vi "Read_Full.vi"(8 "error in (no error)":errorcluster, 10 "Results Array In":dbl[](array[numeric]), 11 "SoftmotionAxis in":refnum<class "SoftmotionAxis.lvclass">) -> (0 "error out":errorcluster, 2 "appended array":dbl[](array[numeric]), 3 "SoftmotionAxis out":refnum<class "SoftmotionAxis.lvclass">)   [LabVIEW 2017, in "SoftmotionAxis.lvclass"]
uses:
  SoftmotionAxis.lvclass
  <resource>/objmgr/nimcai.rc
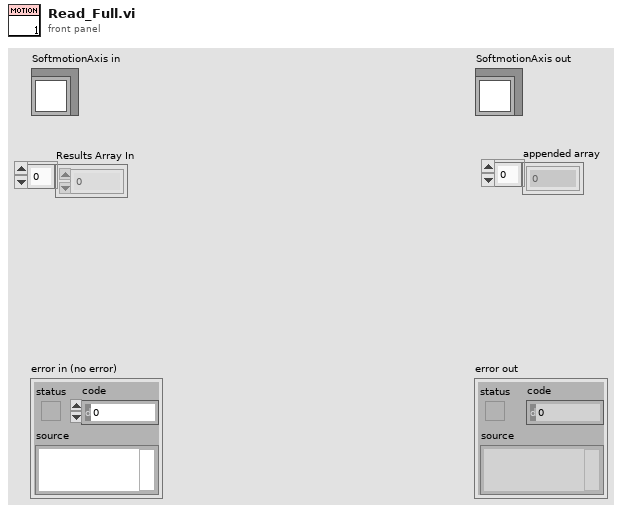
[diagram p1: front panel]
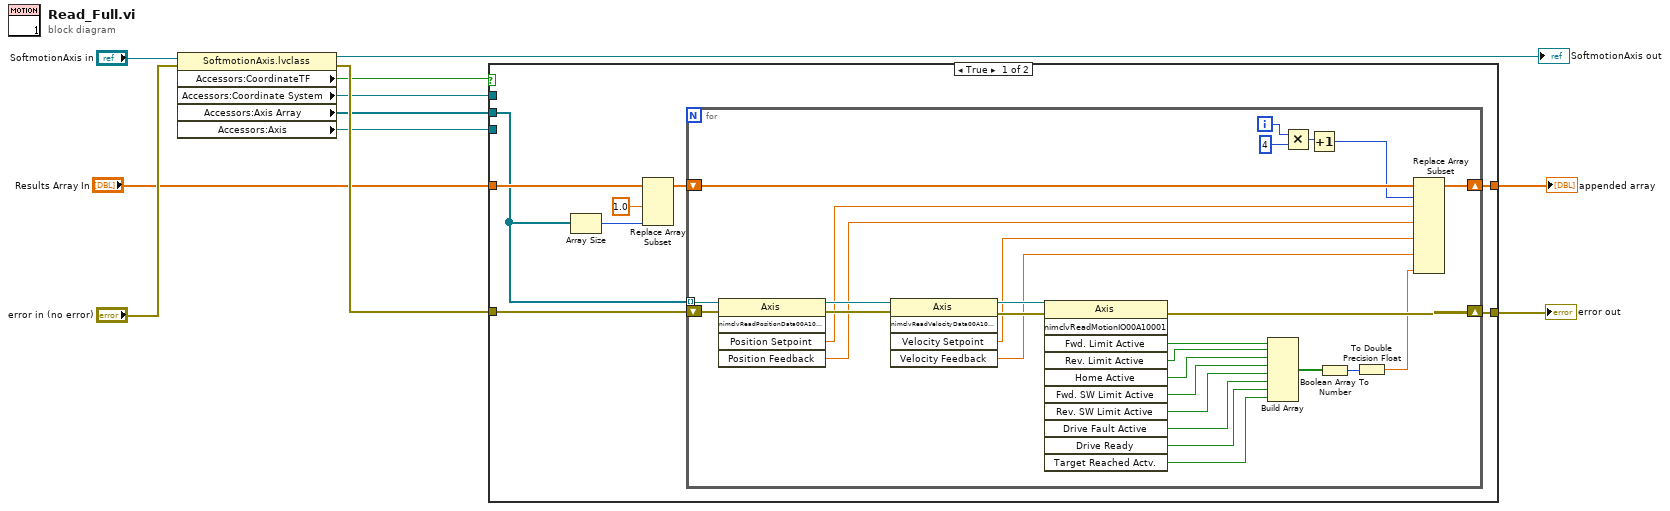
[diagram p0: block diagram]
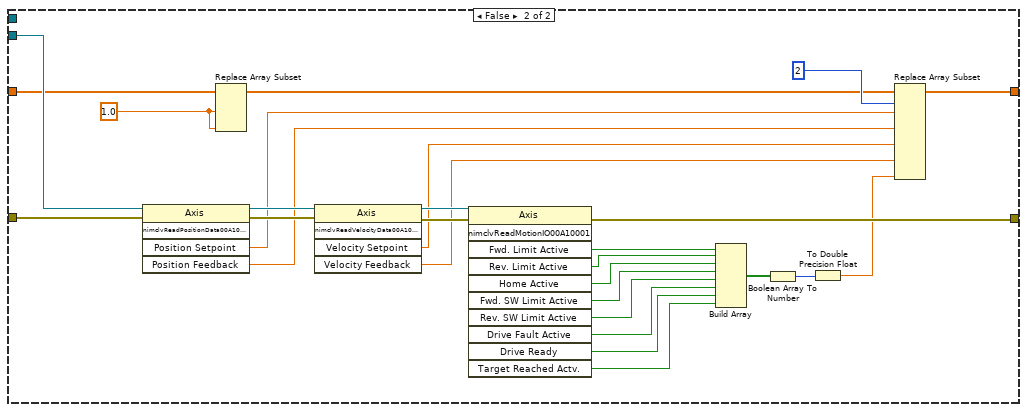
[diagram p2: hidden frame]
diagram:
  n1 = property class="SoftmotionAxis.lvclass"(reference="SoftmotionAxis in", error in="error in (no error)") -> (reference out=→"SoftmotionAxis out":refnum<class "SoftmotionAxis.lvclass">, error out=w11:errorcluster, "Accessors:CoordinateTF"=w9:bool, "Accessors:Coordinate System"=w8:refnum<k21>, "Accessors:Axis Array"=w2:refnum<k21>[], "Accessors:Axis"=w10:refnum<k21>)
  n2 = case shown="True" w9 {
    tunnel: [w17 w57] -> w5
    tunnel: [w19 w64] -> w4
    tunnel: w11 -> [w18 w63]
    tunnel: w10 -> [_ w58]
    tunnel: w8 -> [_ _]
    tunnel: w2 -> [w13 _]
    tunnel: "Results Array In" -> [w15 w50]
    frame True {
      n3 = Array Size(array=w13) -> (size(s)=w12:i32)
      n4 = Replace Array Subset(array=w15, new element #1=1.0 ("new element/subarray"), new element #2=w12) -> (w14:dbl[])  [unwired: 2 in]
      n5 = for {
        shift-right: [w37] -> w19
        shift-left: w18 -> [w36]
        tunnel: w13 -> [w31] mode=indexing
        shift-right: [w26] -> w17
        shift-left: w14 -> [w25]
        i -> [w30]
        n6 = invoke class="Axis" method="nimclvReadPositionData00A10001"(reference=w31, error in=w36) -> (reference out=w35:refnum<k21>, error out=w34:errorcluster, "Position Setpoint"=w28:dbl, "Position Feedback"=w27:dbl)  [unwired: 3 in, 1 out]
        n7 = invoke class="Axis" method="nimclvReadVelocityData00A10001"(reference=w35, error in=w34) -> (reference out=w33:refnum<k21>, error out=w32:errorcluster, "Velocity Setpoint"=w24:dbl, "Velocity Feedback"=w23:dbl)  [unwired: 3 in, 1 out]
        n8 = invoke class="Axis" method="nimclvReadMotionIO00A10001"(reference=w33, error in=w32) -> (error out=w37:errorcluster, "Fwd. Limit Active"=w47:bool, "Rev. Limit Active"=w46:bool, "Home Active"=w45:bool, "Fwd. SW Limit Active"=w44:bool, "Rev. SW Limit Active"=w43:bool, "Drive Fault Active"=w42:bool, "Drive Ready"=w41:bool, "Target Reached Actv."=w40:bool)  [unwired: 9 in, 2 out]
        n9 = Build Array(w47, w46, w45, w44, w43, w42, w41, w40) -> (w39:bool[])
        n10 = Multiply(x=w30, y=4) -> (x*y=w21:i32)
        n11 = Increment(x=w21) -> (x+1=w20:i32)
        n12 = Boolean Array To Number(Boolean array=w39) -> (number=w38:u32)
        n13 = To Double Precision Float(number=w38) -> (double precision float=w22:dbl)
        n14 = Replace Array Subset(array=w25, new element #1=w28, index #1=w20, new element #2=w27, new element #3=w24, new element #4=w23, new element #5=w22) -> (w26:dbl[])  [unwired: 4 in]
      }
    }
    frame False {
      w48 = 1.0 ("new element/subarray")
      n15 = invoke class="Axis" method="nimclvReadPositionData00A10001"(reference=w58, error in=w63) -> (reference out=w62:refnum<k21>, error out=w61:errorcluster, "Position Setpoint"=w55:dbl, "Position Feedback"=w56:dbl)  [unwired: 3 in, 1 out]
      n16 = Replace Array Subset(array=w50, new element #1=w48, new element #2=w48) -> (w49:dbl[])  [unwired: 2 in]
      n17 = invoke class="Axis" method="nimclvReadVelocityData00A10001"(reference=w62, error in=w61) -> (reference out=w60:refnum<k21>, error out=w59:errorcluster, "Velocity Setpoint"=w52:dbl, "Velocity Feedback"=w53:dbl)  [unwired: 3 in, 1 out]
      n18 = invoke class="Axis" method="nimclvReadMotionIO00A10001"(reference=w60, error in=w59) -> (error out=w64:errorcluster, "Fwd. Limit Active"=w74:bool, "Rev. Limit Active"=w73:bool, "Home Active"=w72:bool, "Fwd. SW Limit Active"=w71:bool, "Rev. SW Limit Active"=w70:bool, "Drive Fault Active"=w69:bool, "Drive Ready"=w68:bool, "Target Reached Actv."=w67:bool)  [unwired: 9 in, 2 out]
      n19 = Build Array(w74, w73, w72, w71, w70, w69, w68, w67) -> (w66:bool[])
      n20 = Boolean Array To Number(Boolean array=w66) -> (number=w65:u32)
      n21 = To Double Precision Float(number=w65) -> (double precision float=w54:dbl)
      n22 = Replace Array Subset(array=w49, new element #1=w55, index #1=2 ("index"), new element #2=w56, new element #3=w52, new element #4=w53, new element #5=w54) -> (w57:dbl[])  [unwired: 4 in]
    }
  }
  "error out" <- w4
  "appended array" <- w5
